vi "nirviSaturationSubtract.vi"(9 "x":i16, 13 "y":i16) -> (10 "x-y":i16, 18 "overflow":bool)   [LabVIEW 2017]
doc: "Computes the difference between the inputs with configurable overflow handling and an optional overflow output terminal."
panel:
  in  "operation":u16(ring)=1 items=["Add", "Sub", "Mult"]
  in  "Overflow terminal":bool
  in  "Lower Limit":i16=-128
  in  "Upper Limit":i16=127
  in  "Saturation":bool=TRUE
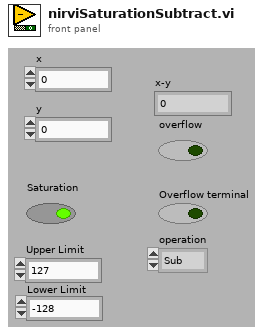
[diagram p1: front panel]
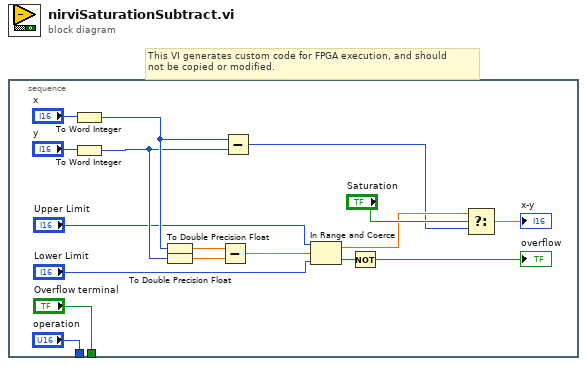
[diagram p0: block diagram]
diagram:
  # "This VI generates custom code for FPGA execution, and should\nnot be copied or modified."
  n1 = stacked-sequence {
    tunnel: ["Overflow terminal"] -> _
    tunnel: ["operation"] -> _
    frame #0 {
      n2 = To Word Integer(number="x") -> (16bit integer=w15:i16)
      n3 = To Word Integer(number="y") -> (16bit integer=w14:i16)
      n4 = To Double Precision Float(number=w15) -> (double precision float=w7:dbl)
      n5 = To Double Precision Float(number=w14) -> (double precision float=w8:dbl)
      n6 = Subtract(x=w7, y=w8) -> (x-y=w5:dbl)
      n7 = Subtract(x=w15, y=w14) -> (x-y=w3:i16)
      n8 = In Range and Coerce(upper limit="Upper Limit", x=w5, lower limit="Lower Limit") -> (coerced(x)=w4:dbl, In Range?=w6:bool)
      n9 = Not(x=w6) -> (.not. x?=→"overflow":bool)
      n10 = Select(t=w4, s="Saturation", f=w3) -> (s? t:f=→"x-y":dbl)
    }
  }
